vi "readFromXML.vi"(8 "error in (no error)":errorcluster, 10 "XML in":string, 11 "Wrapnum in":refnum<class "Wrapnum.lvclass">) -> (0 "error out":errorcluster, 3 "Wrapnum out":refnum<class "Wrapnum.lvclass">)   [LabVIEW 2010, in "TCS.lvlib" / "TCSDataDefinitions.lvlib" / "TCSCommand.lvlib" / "Wrapnum.lvclass"]
uses:
  Wrapnum.lvclass
  Wrapnum.lvclass/Wrapnum.ctl
  Common/XML/XML.lvlib
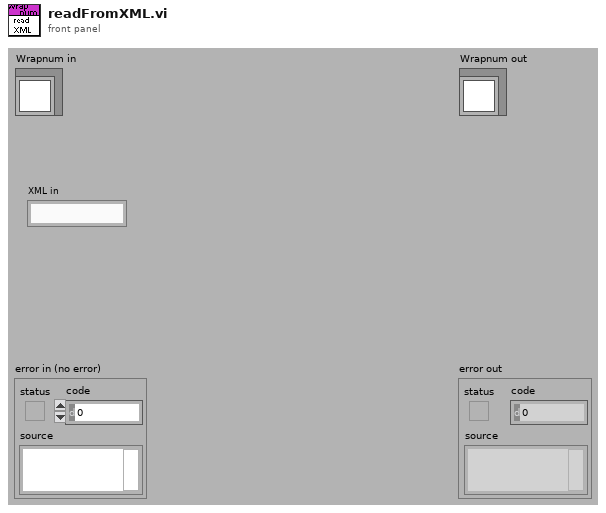
[diagram p1: front panel]
types:
  T1 = typedef "TCS.lvlib/TCSDataDefinitions.lvlib/TCSCommand.lvlib/WrapnumTypes.ctl" = enum16{"-1", "0", "1"}
  T2 = typedef "XML.lvlib/XML element list.ctl" = T3[]
  T3 = typedef "XML.lvlib/XML element.ctl" = cluster{"name":string, "contents":string}
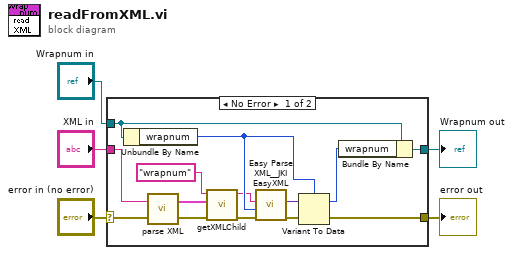
[diagram p0: block diagram]
diagram:
  n1 = case shown="No Error" "error in (no error)" {
    selector: "error in (no error)" -> [w9 w21]
    tunnel: [w13 w21] -> w4
    tunnel: [w14 w20] -> w2
    tunnel: "Wrapnum in" -> [w15 w20]
    tunnel: "XML in" -> [w10 _]
    frame No Error {
      n2 = Unbundle By Name(w15) -> ("wrapnum"=w17:T1)
      n3 = call "parse XML.vi"("error in (no error)"=w9, "XMLString in"=w10) -> ("error out"=w11:errorcluster, "XML element list out"=w12:T2)
      n4 = call "getXMLChild.vi"("error in (no error)"=w11, "XML element list in"=w12, "ChildName"="wrapnum") -> ("error out"=w8:errorcluster, "XML content string out"=w7:string)  [unwired: 6 in, 1 out]
      n5 = call <vilib>:"Easy Parse XML__JKI EasyXML.vi"("error in (no error)"=w8, "LabVIEW Data (Type)"=w17, "XML String"=w7) -> ("error out"=w19:errorcluster, "LabVIEW Data"=w18:variant)  [unwired: 7 out]
      n6 = Variant To Data(error in=w19, Variant=w18, type=w17) -> (error out=w13:errorcluster, data=w16:T1)
      n7 = Bundle By Name(cluster=w15, "wrapnum"=w16) -> (w14:refnum<class "Wrapnum.lvclass">)
    }
    frame Error {
    }
  }
  "error out" <- w4
  "Wrapnum out" <- w2
